vi "Detect Chassis Modules.vi"(8 "error in":errorcluster, 11 "Controller in":refnum<class "Controller.lvclass">) -> (0 "error out":errorcluster, 3 "Controller out":refnum<class "Controller.lvclass">)   [LabVIEW 2015, in "SMI.lvlib" / "Chassis.lvclass"]
uses:
  Chassis.lvclass
  Controller/Controller.lvclass
  Controller/Controller.lvclass/Controller.ctl
  C Series Module/C Series Module.lvclass
  PXI Module/PXI Module.lvclass
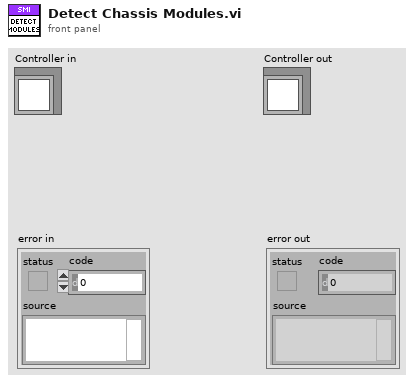
[diagram p1: front panel]
types:
  T1 = typedef "SMI.lvlib/Controller.lvclass/DeviceInformation.ctl" = cluster{"Resource":string, "Device Class":string, "System Start Time":timestamp, "Current Time":timestamp, "Time Zone":string, "Firmware Revision":string, "Image Title":string, "Image Version":string, "System Status":string, "Credential type":enum16{"None/Unlocked", "FTP Password", "NIAuth Credentials"}, "User Added":bool}
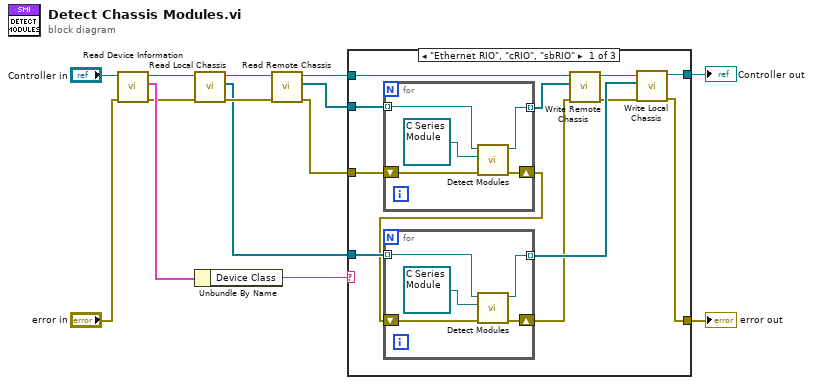
[diagram p0: block diagram]
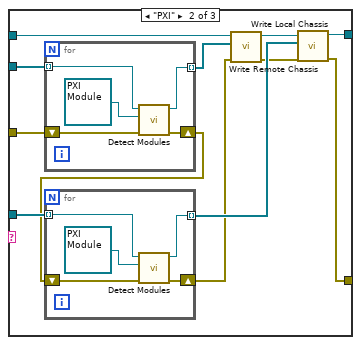
[diagram p2: hidden frame]
diagram:
  n1 = call "Read Device Information.vi"("error in (no error)"="error in", "Controller in"="Controller in") -> ("error out"=w6:errorcluster, "Device Information"=w12:T1, "Controller out"=w8:refnum<class "Controller.lvclass">)  [unwired: 7 in]
  n2 = call "Read Local Chassis.vi"("error in (no error)"=w6, "Controller in"=w8) -> ("error out"=w7:errorcluster, "Local Chassis"=w2:refnum<class "Chassis.lvclass">[], "Controller out"=w9:refnum<class "Controller.lvclass">)  [unwired: 7 in]
  n3 = Unbundle By Name(w12) -> ("Device Class"=w11:string)
  n4 = call "Read Remote Chassis.vi"("error in (no error)"=w7, "Controller in"=w9) -> ("error out"=w5:errorcluster, "Remote Chassis"=w3:refnum<class "Chassis.lvclass">[], "Controller out"=w4:refnum<class "Controller.lvclass">)  [unwired: 7 in]
  n5 = case shown="\"Ethernet RIO\", \"cRIO\", \"sbRIO\"" w11 {
    tunnel: [w15 w37 w60] -> w10
    tunnel: w5 -> [w19 w41 w60]
    tunnel: w2 -> [w26 w48 _]
    tunnel: w3 -> [w25 w47 _]
    tunnel: w4 -> [w24 w46 w59]
    tunnel: [w22 w44 w59] -> w1
    frame "Ethernet RIO", "cRIO", "sbRIO" {
      n6 = for {
        tunnel: w25 -> [w30] mode=indexing
        tunnel: [w29] -> w21 mode=indexing
        shift-right: [w28] -> w18
        shift-left: w19 -> [w27]
        n7 = call-dynamic "Detect Modules.vi"("error in"=w27, "C Series Module in"=refnum<class "C Series Module.lvclass"> refnum ("SMI.lvlib:C Series Module.lvclass"), "Chassis in"=w30) -> ("error out"=w28:errorcluster, "Chassis out"=w29:refnum<class "Chassis.lvclass">)  [unwired: 6 in, 1 out]
      }
      n8 = for {
        tunnel: w26 -> [w35] mode=indexing
        tunnel: [w34] -> w20 mode=indexing
        shift-right: [w33] -> w16
        shift-left: w18 -> [w32]
        n9 = call-dynamic "Detect Modules.vi"("error in"=w32, "C Series Module in"=refnum<class "C Series Module.lvclass"> refnum ("SMI.lvlib:C Series Module.lvclass"), "Chassis in"=w35) -> ("error out"=w33:errorcluster, "Chassis out"=w34:refnum<class "Chassis.lvclass">)  [unwired: 6 in, 1 out]
      }
      n10 = call "Write Remote Chassis.vi"("error in (no error)"=w16, "Remote Chassis"=w21, "Controller in"=w24) -> ("error out"=w17:errorcluster, "Controller out"=w23:refnum<class "Controller.lvclass">)  [unwired: 7 in]
      n11 = call "Write Local Chassis.vi"("error in (no error)"=w17, "Local Chassis"=w20, "Controller in"=w23) -> ("error out"=w15:errorcluster, "Controller out"=w22:refnum<class "Controller.lvclass">)  [unwired: 7 in]
    }
    frame "PXI" {
      n12 = for {
        tunnel: w47 -> [w52] mode=indexing
        tunnel: [w51] -> w43 mode=indexing
        shift-right: [w50] -> w40
        shift-left: w41 -> [w49]
        n13 = call-dynamic "Detect Modules.vi"("error in"=w49, "PXI Module in"=refnum<class "PXI Module.lvclass"> refnum ("SMI.lvlib:PXI Module.lvclass"), "Chassis in"=w52) -> ("error out"=w50:errorcluster, "Chassis out"=w51:refnum<class "Chassis.lvclass">)  [unwired: 6 in, 1 out]
      }
      n14 = for {
        tunnel: w48 -> [w57] mode=indexing
        tunnel: [w56] -> w42 mode=indexing
        shift-right: [w55] -> w38
        shift-left: w40 -> [w54]
        n15 = call-dynamic "Detect Modules.vi"("error in"=w54, "PXI Module in"=refnum<class "PXI Module.lvclass"> refnum ("SMI.lvlib:PXI Module.lvclass"), "Chassis in"=w57) -> ("error out"=w55:errorcluster, "Chassis out"=w56:refnum<class "Chassis.lvclass">)  [unwired: 6 in, 1 out]
      }
      n16 = call "Write Remote Chassis.vi"("error in (no error)"=w38, "Remote Chassis"=w43, "Controller in"=w46) -> ("error out"=w39:errorcluster, "Controller out"=w45:refnum<class "Controller.lvclass">)  [unwired: 7 in]
      n17 = call "Write Local Chassis.vi"("error in (no error)"=w39, "Local Chassis"=w42, "Controller in"=w45) -> ("error out"=w37:errorcluster, "Controller out"=w44:refnum<class "Controller.lvclass">)  [unwired: 7 in]
    }
    frame Default {
    }
  }
  "error out" <- w10
  "Controller out" <- w1
